vi "resolve vi references.vi"(11 "remaining string":string) -> (2 "VI name":string, 3 "VI out":refnum<vi>)   [LabVIEW 2013, in "UI Reference configuration.lvclass"]
uses:
  UI Reference configuration.lvclass
  <vilib>/NI/Tag Bus Module Framework/root configuration/TBM configuration.lvclass
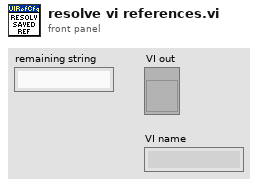
[diagram p1: front panel]
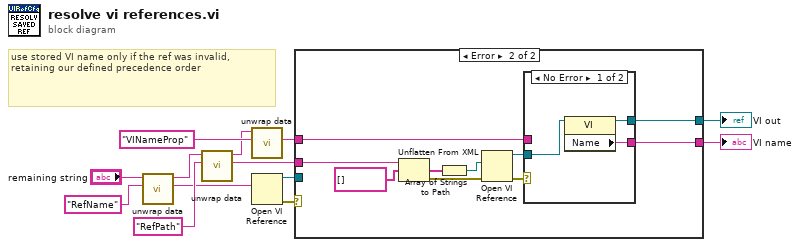
[diagram p0: block diagram]
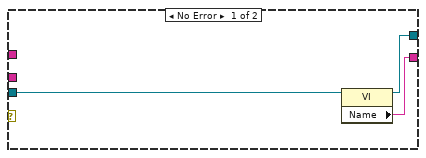
[diagram p2: hidden frame]
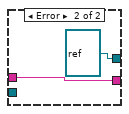
[diagram p3: hidden frame]
diagram:
  # "use stored VI name only if the ref was invalid, retaining our defined precedence order"
  n1 = call <vilib>:"unwrap data.vi"("identifier"="RefName" ("additional identifier"), "data to unwrap"="remaining string") -> ("unwrapped data"=w6:string, "remaining string"=w11:string)  [unwired: 8 in]
  n2 = call <vilib>:"unwrap data.vi"("identifier"="RefPath" ("additional identifier"), "data to unwrap"=w11) -> ("unwrapped data"=w7:string, "remaining string"=w12:string)  [unwired: 8 in]
  n3 = call <vilib>:"unwrap data.vi"("identifier"="VINameProp" ("additional identifier"), "data to unwrap"=w12) -> ("unwrapped data"=w1:string)  [unwired: 8 in, 1 out]
  n4 = Open VI Reference(vi path=w6) -> (vi reference=w3:refnum<vi>, error out=w5:errorcluster)  [unwired: 5 in]
  n5 = case shown="Error" w5 {
    tunnel: w7 -> [_ w22]
    tunnel: [w15 w20] -> w4
    tunnel: w3 -> [w16 _]
    tunnel: [w14 w17] -> w2
    tunnel: w1 -> [_ w18]
    frame No Error {
      n6 = property class="VI"(reference=w16) -> (reference out=w15:refnum<vi>, "Name"=w14:string)  [unwired: 1 in, 1 out]
    }
    frame Error {
      n7 = Unflatten From XML(xml string=w22, type=string[] [] ("array of strings")) -> (value=w25:string[], error out=w24:errorcluster)  [unwired: 1 in]
      n8 = Array of Strings to Path(0:w25) -> (2:w23:path)  [unwired: 1 in]
      n9 = Open VI Reference(vi path=w23, error in (no error)=w24) -> (vi reference=w19:refnum<vi>, error out=w21:errorcluster)  [unwired: 4 in]
      n10 = case shown="No Error" w21 {
        tunnel: [w28 refnum<vi> refnum ("vi reference")] -> w20
        tunnel: w19 -> [w29 _]
        tunnel: w18 -> [_ w30]
        tunnel: [w27 w30] -> w17
        frame No Error {
          n11 = property class="VI"(reference=w29) -> (reference out=w28:refnum<vi>, "Name"=w27:string)  [unwired: 1 in, 1 out]
        }
        frame Error {
        }
      }
    }
  }
  "VI out" <- w4
  "VI name" <- w2
